vi "Application user.lib.vi"(8 "error in":errorcluster) -> (0 "error out":errorcluster, 3 "path out":path)   [LabVIEW 2019, in "Control Experiment.lvclass"]
uses:
  <vilib>/Utility/sysdir.llb/System Directory Type.ctl
  Control Experiment.lvclass
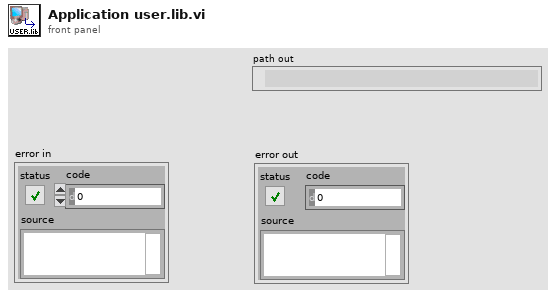
[diagram p1: front panel]
types:
  T1 = typedef "System Directory Type.ctl" = i32
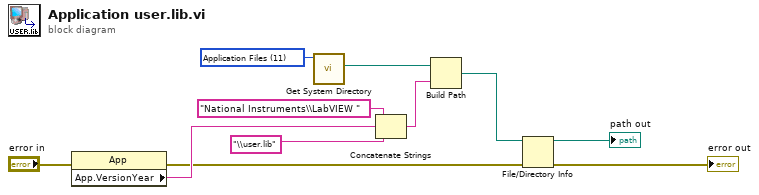
[diagram p0: block diagram]
diagram:
  w11 = T1 11 items=["User Home"=0, "User Desktop"=1, "User Documents"=2, "User Application Data"=3, "User Preferences"=4, "User Temporary"=5, "Public Documents"=6, "Public Application Data"=7, "Public Preferences"=8, "Public Cache"=13, "System Core Libraries"=9, "System Installed Libraries"=10, "Application Files"=11, "Boot Volume Root"=12] ("system directory type")
  n1 = property class="App"(error in="error in") -> (error out=w4:errorcluster, "App.VersionYear"=w10:string)  [unwired: 1 in, 1 out]
  n2 = call <vilib>:"Get System Directory.vi"("system directory type"=w11) -> ("system directory"=w9:path)  [unwired: 10 in]
  n3 = Concatenate Strings("National Instruments\\LabVIEW " ("string"), w10, "\\user.lib" ("string")) -> (w2:string)
  n4 = Build Path(base path=w9, name or relative path=w2) -> (appended path=w1:path)
  n5 = File/Directory Info(path=w1, error in=w4) -> (path out=→"path out":path, error out=→"error out":errorcluster)  [unwired: 5 out]
